vi "Different Types.vi"() -> ()   [LabVIEW 2017, in "Transparent Assertions.Tests.lvlib" / "Assert Not Same Type.lvlib"]
uses:
  Assert Not Same Type.lvlib
  src/Transparent Assertions/Transparent Assertions.lvlib
panel:
  out "error out":errorcluster
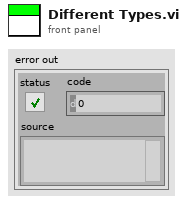
[diagram p1: front panel]
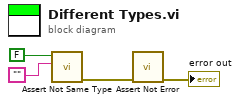
[diagram p0: block diagram]
diagram:
  n1 = call "Assert Not Same Type.vi"("Second"="", "First"=FALSE) -> ("error out"=w3:errorcluster)  [unwired: 9 in]
  n2 = call "Assert Not Error.vi"("error in (no error)"=w3) -> ("error out"=→"error out":errorcluster)  [unwired: 10 in]
